vi "RS.vi"(2 "S":bool, 3 "R":bool) -> (0 "not Q":bool, 1 "Q":bool)   [LabVIEW 2012]
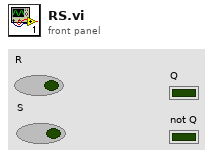
[diagram p1: front panel]
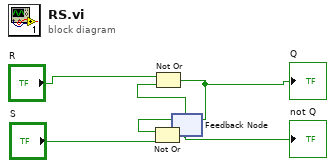
[diagram p0: block diagram]
diagram:
  n1 = feedback #1() -> (w2:bool)  [unwired: 1 in]
  n2 = Not Or(1:"S", 2:w2) -> (0:w3:bool)
  "not Q" <- w3
  n3 = Not Or(1:w3, 2:"R") -> (0:w1:bool)
  "Q" <- w1
  n4 = feedback-in #1(w1) -> ()
